vi "Write Write_.vi"(8 "error in (no error)":errorcluster, 10 "Write?":bool, 11 "Update Write Ringdowns MSG in":refnum<class "Update Write Ringdowns MSG.lvclass">) -> (0 "error out":errorcluster, 3 "Update Write Ringdowns MSG out":refnum<class "Update Write Ringdowns MSG.lvclass">)   [LabVIEW 2014, in "eCRDS Library.lvlib" / "Update Write Ringdowns MSG.lvclass"]
uses:
  Update Write Ringdowns MSG.lvclass
  Update Write Ringdowns MSG.lvclass/Update Write Ringdowns MSG.ctl
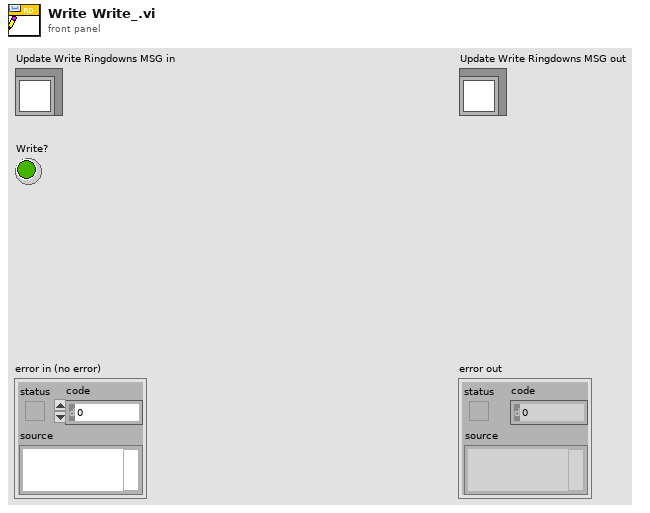
[diagram p1: front panel]
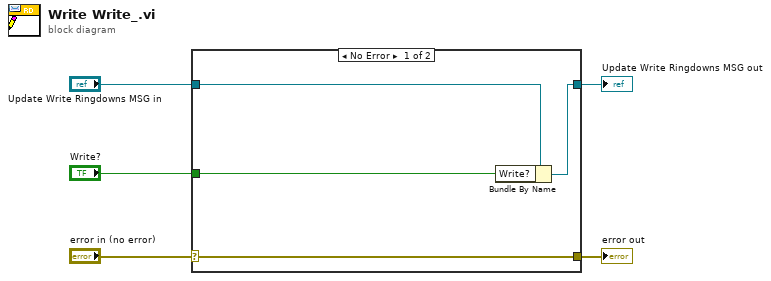
[diagram p0: block diagram]
diagram:
  n1 = case shown="No Error" "error in (no error)" {
    selector: "error in (no error)" -> [w9 w10]
    tunnel: [w9 w10] -> w4
    tunnel: [w7 w11] -> w2
    tunnel: "Update Write Ringdowns MSG in" -> [w8 w11]
    tunnel: "Write?" -> [w6 _]
    frame No Error {
      n2 = Bundle By Name(cluster=w8, "Write?"=w6) -> (w7:refnum<class "Update Write Ringdowns MSG.lvclass">)
    }
    frame Error {
    }
  }
  "error out" <- w4
  "Update Write Ringdowns MSG out" <- w2
